vi "util.DO.ToString.vi"(9 "error in":errorcluster, 10 "output cluster":cluster{"state":bool, "timeoutSeconds":u16}) -> (1 "error IO":errorcluster, 2 "initial string":string="1:3")   [LabVIEW 2024]
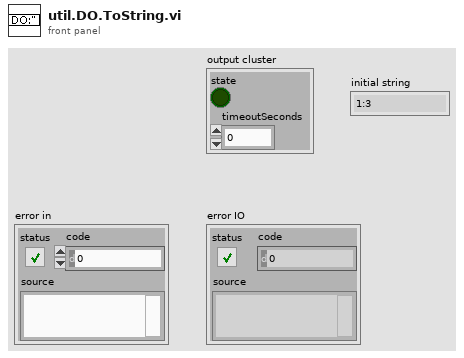
[diagram p1: front panel]
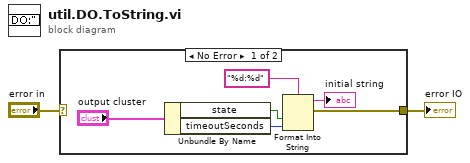
[diagram p0: block diagram]
diagram:
  n1 = case shown="No Error" "error in" {
    selector: "error in" -> [_ w9]
    tunnel: [w3 w9] -> w1
    frame No Error {
      n2 = Unbundle By Name("output cluster") -> ("state"=w6:bool, "timeoutSeconds"=w5:u16)
      n3 = Format Into String(format string="%d:%d", w6, w5) -> (resulting string=→"initial string":string, error out=w3:errorcluster)  [unwired: 2 in]
    }
    frame Error {
    }
  }
  "error IO" <- w1
